vi "zc init log with callback.vi"(8 "error in (no error)":errorcluster, 10 "callback":cluster{"_context":u64, "_call":u64}, 11 "min_severity":u32(ring) items=["ZC_LOG_SEVERITY_TRACE", "ZC_LOG_SEVERITY_DEBUG", "ZC_LOG_SEVERITY_INFO", "ZC_LOG_SEVERITY_WARN", "ZC_LOG_SEVERITY_ERROR"]) -> (0 "error out":errorcluster, 2 "callback out":cluster{"_context":u64, "_call":u64})   [LabVIEW 2021, in "zenohc.lvlib"]
doc: "void zc_init_log_with_callback(enum zc_log_severity_t min_severity,\n struct zc_moved_closure_log_t *callback);"
uses:
  zenohc.lvlib
  zenohc.dll
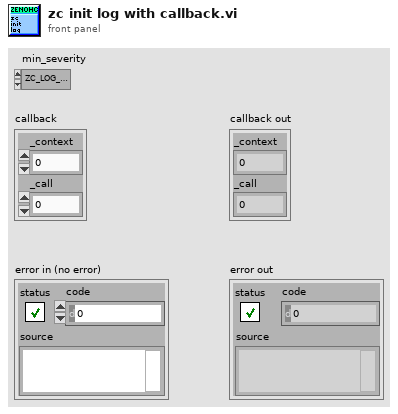
[diagram p1: front panel]
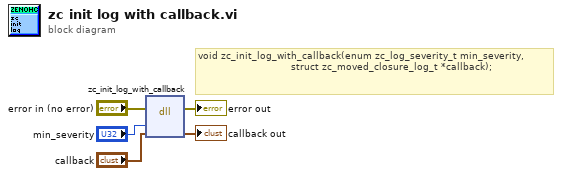
[diagram p0: block diagram]
diagram:
  # "void zc_init_log_with_callback(enum zc_log_severity_t min_severity,\n                               struct zc_moved_closure_log_t *callback);"
  n1 = dll-call lib="D:/dev/zenoh_labview/zenohc/zenohc.*" fn="zc_init_log_with_callback"(error in="error in (no error)", "min_severity"="min_severity", "callback"="callback") -> (error out=→"error out":errorcluster, "callback"=→"callback out":cluster{"_context":u64, "_call":u64})  [unwired: 4 in, 1 out]
